vi "指令生成.vi"(9 "伪装\\解密":bool, 11 "路径":path) -> (3 "指令":string)   [LabVIEW 2009]
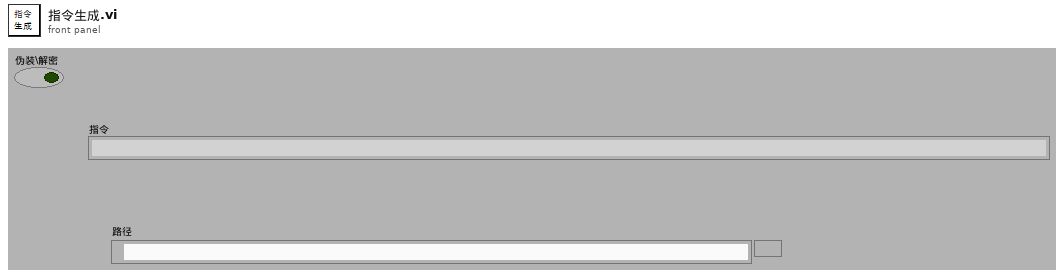
[diagram p1: front panel]
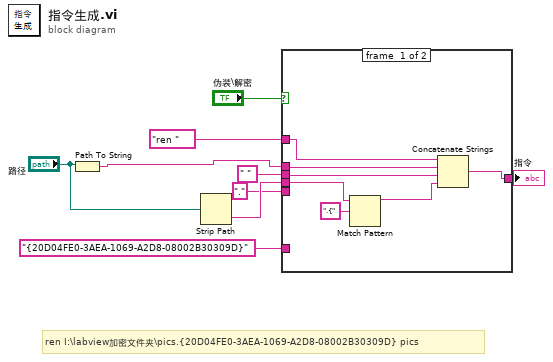
[diagram p0: block diagram]
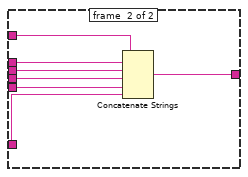
[diagram p2: hidden frame]
diagram:
  # "ren I:\\labview加密文件夹\\pics.{20D04FE0-3AEA-1069-A2D8-08002B30309D} pics"
  n1 = Path To String(path="路径") -> (string=w1:string)
  n2 = Strip Path(path="路径") -> (name=w6:string)  [unwired: 1 out]
  n3 = case shown="假" "伪装\\解密" {
    tunnel: "ren " -> [w15 w23]
    tunnel: w1 -> [w14 w22]
    tunnel: " " ("字符串") -> [w13 w21]
    tunnel: w6 -> [w12 w20]
    tunnel: "." ("字符串") -> [_ w19]
    tunnel: "{20D04FE0-3AEA-1069-A2D8-08002B30309D}" ("字符串") -> [_ w18]
    tunnel: [w16 w17] -> w2
    frame #0 {
      n4 = Match Pattern(string=w12, regular expression=".{" ("正则表达式")) -> (before substring=w11:string)  [unwired: 1 in, 3 out]
      n5 = Concatenate Strings(w15, w14, w13, w11) -> (w16:string)
    }
    frame #1 {
      n6 = Concatenate Strings(w23, w22, w21, w20, w19, w18) -> (w17:string)
    }
  }
  "指令" <- w2
